vi "Read Logger.vi"(8 "error in (no error)":errorcluster, 11 "Word Log Producer in":refnum<class "Word Log Producer.lvclass">=refnum) -> (0 "error out":errorcluster, 2 "Logger":refnum<class "Word Logger Interface.lvclass">, 3 "Word Log Producer out":refnum<class "Word Log Producer.lvclass">)   [LabVIEW 2024]
uses:
  Word Log Producer.lvclass
  Word Logger Interface/Word Logger Interface.lvclass
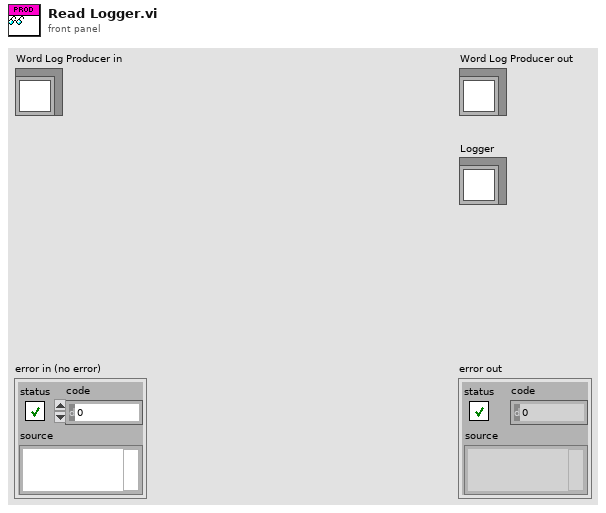
[diagram p1: front panel]
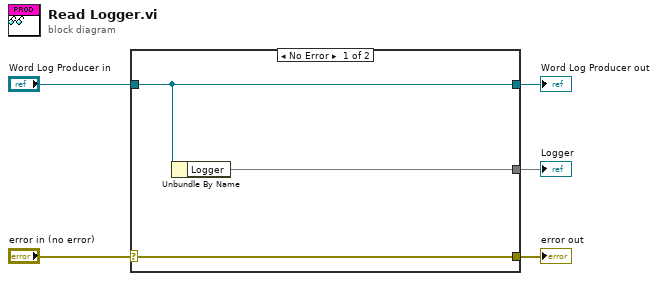
[diagram p0: block diagram]
diagram:
  n1 = case shown="No Error" "error in (no error)" {
    selector: "error in (no error)" -> [w8 w9]
    tunnel: [w8 w9] -> w4
    tunnel: [w7 w10] -> w2
    tunnel: "Word Log Producer in" -> [w7 w10]
    tunnel: [w6 _] -> w1
    frame No Error {
      n2 = Unbundle By Name(w7) -> ("Logger"=w6)
    }
    frame Error {
    }
  }
  "error out" <- w4
  "Word Log Producer out" <- w2
  "Logger" <- w1
